vi "Clear Buffer.vi"(8 "error in (no error)":errorcluster, 9 "offset (0)":u64 format="%d bytes", 10 "length (-1: rest)":i64=-1 format="%d bytes", 11 "Buffer in":refnum<class "Buffer.lvclass">) -> (0 "error out":errorcluster, 3 "Buffer out":refnum<class "Buffer.lvclass">)   [LabVIEW 2017, in "DSF Core.lvlib" / "Buffer.lvclass"]
uses:
  Buffer.lvclass
  C:/Git/DSF/LabVIEW-Memory/Source/Classes/Pointer/Pointer.lvclass
  LabVIEW-Memory/Source/Classes/Pointer/Pointer.lvclass
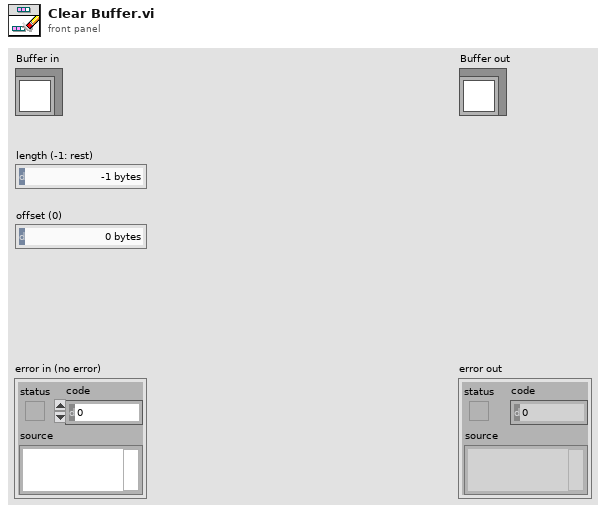
[diagram p1: front panel]
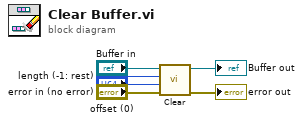
[diagram p0: block diagram]
diagram:
  n1 = call "Clear.vi"("error in (no error)"="error in (no error)", "offset (0)"="offset (0)", "length (-1: rest)"="length (-1: rest)", "Pointer in"="Buffer in") -> ("error out"=→"error out":errorcluster, "Pointer out"=→"Buffer out":refnum<class "Buffer.lvclass">)  [unwired: 6 in]
